vi "Add Topic Subscriber.vi"(8 "error in (no error)":errorcluster, 10 "Subscription Policy":T1, 11 "Topic in":refnum<class "Topic.lvclass">) -> (0 "error out":errorcluster, 3 "Topic out":refnum<class "Topic.lvclass">)   [LabVIEW 2020, in "Mediator.lvlib" / "Topic.lvclass"]
doc: "添加主题订阅者"
uses:
  Topic.lvclass
  IMediator/ISubscriptionPolicy/ISubscriptionPolicy Reference.ctl
  IMediator/ISubscriptionPolicy/ISubscriptionPolicy.lvclass
  Topic.lvclass/Topic.ctl
  IMediator/ISubscriptionPolicy/ISubscriptionPolicy.lvclass/ISubscriptionPolicy.ctl
  <vilib>/Utility/error.llb/Trim Whitespace.vi
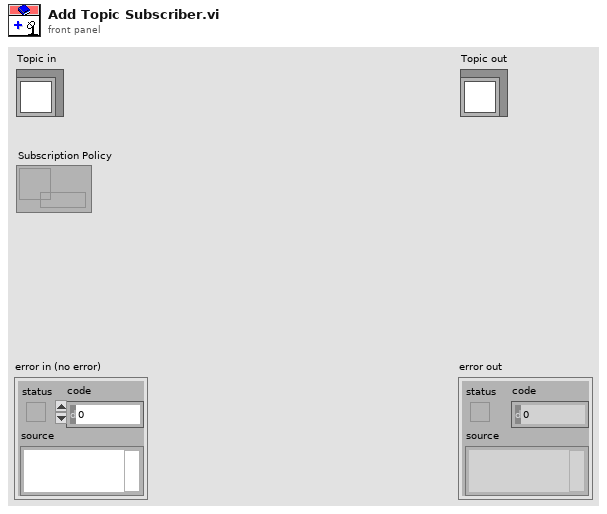
[diagram p1: front panel]
types:
  T1 = typedef "IMediator.lvlib/ISubscriptionPolicy.lvclass/ISubscriptionPolicy Reference.ctl" = refnum<data-value>
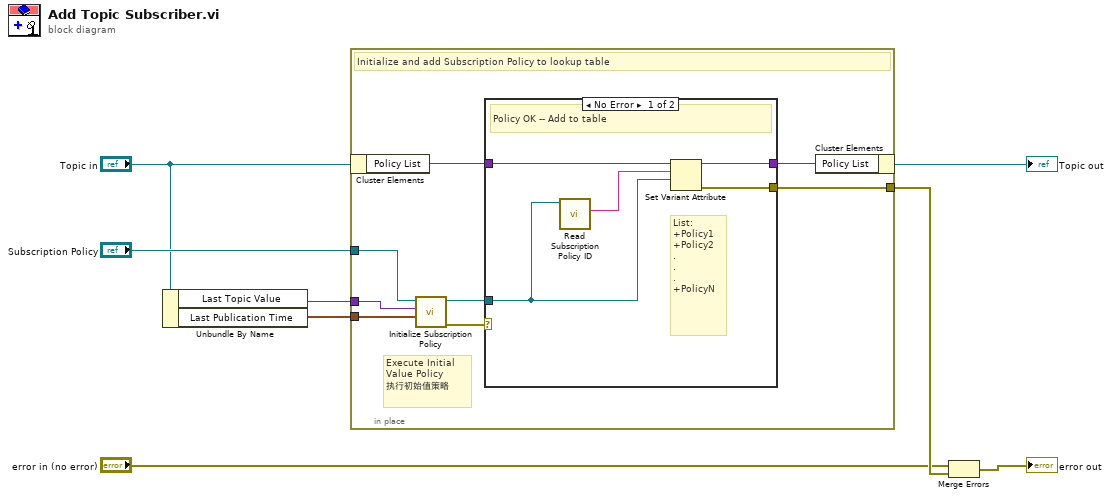
[diagram p0: block diagram]
diagram:
  n1 = Unbundle By Name("Topic in") -> ("Last Topic Value"=w4:variant, "Last Publication Time"=w3:timestamp)
  n2 = in-place {
    in-place-border: [w14] -> w8
    in-place-border: "Subscription Policy" -> [w10]
    in-place-border: w4 -> [w13]
    in-place-border: w3 -> [w11]
    # "Execute Initial\nValue Policy\n执行初始值策略"
    # "Initialize and add Subscription Policy to lookup table"
    n3 = in-place-cluster #1("Topic in") -> ("Policy List"=w16:variant)
    n4 = call "Initialize Subscription Policy.vi"("Last Publish Time"=w11, "Last Topic Value"=w13, "Subscription Policy"=w10) -> ("Error Out (Unsubscribe?)"=w12:errorcluster, "Subscription Policy Out"=w9:T1)  [unwired: 7 in]
    n5 = case shown="No Error" w12 {
      tunnel: w16 -> [w19 w22]
      tunnel: [w21 w22] -> w15
      tunnel: [w20 _] -> w14
      tunnel: w9 -> [w17 _]
      frame No Error {
        # "List:\n+Policy1\n+Policy2\n.\n.\n.\n+PolicyN"
        # "Policy OK -- Add to table"
        n6 = call "Read Subscription Policy ID.vi"("SubscriptionPolicy"=w17) -> ("Policy ID"=w18:string)  [unwired: 10 in]
        n7 = Set Variant Attribute(Variant=w19, name=w18, value=w17) -> (Variant out=w21:variant, error out=w20:errorcluster)  [unwired: 1 in, 1 out]
      }
      frame Error {
        # "Policy is not valid --\nDo not add to table"
        # "A rough start -- Discard request"
      }
    }
    n8 = in-place-cluster #1("Policy List"=w15) -> (→"Topic out":refnum<class "Topic.lvclass">)
  }
  n9 = Merge Errors("error in (no error)", w8) -> (→"error out":errorcluster)
